vi "GameMode.vi"() -> ()   [LabVIEW 2017]
doc: "SubVI criada para mostrar um pop up para o usuário no caso de jogo multiplayer. O usuário poderá escolher entre as opções Um computador, em que os dois jogadores utilizam a mesma máquina, ou Pela Rede, em que cada computador joga por uma máquina."
panel:
  in  "Rede":bool
  in  "Computador":bool
  # "Qual modo de jogo?"
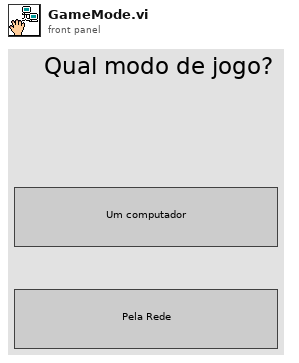
[diagram p1: front panel]
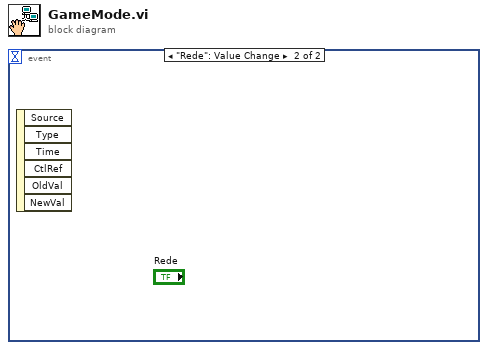
[diagram p0: block diagram]
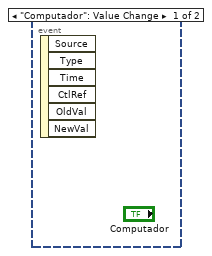
[diagram p2: hidden frame]
diagram:
  n1 = event shown="[1] \"Rede\": Value Change" {
    selector: _ -> [_ _]
    dyn-events: _ -> [_ _]
    timeout: _ -> [_ _]
    event "Computador": Value Change {
      n2 = event-data() -> ()  [unwired: 1 in, 6 out]
    }
    event "Rede": Value Change {
      n3 = event-data() -> ()  [unwired: 1 in, 6 out]
    }
  }
